vi "_FPGA_Driver_DIO_v1_3.vi"(10 "DO":u8) -> (2 "DI":u8)   [LabVIEW 2018]
uses:
  <vilib>/rvi/eio/common/nirviEmuTemplateMethod_errors.vi
  <vilib>/eio/EIONode/EIONode.xnode
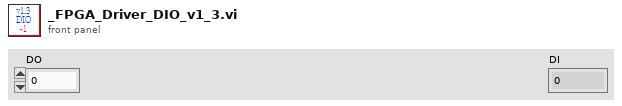
[diagram p1: front panel]
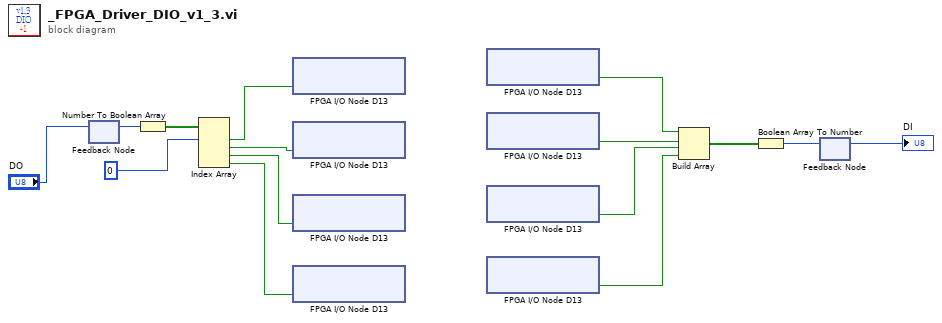
[diagram p0: block diagram]
diagram:
  n1 = feedback-in #1("DO") -> ()
  n2 = feedback #1() -> (w10:u8)  [unwired: 1 in]
  n3 = Number To Boolean Array(number=w10) -> (Boolean array=w14:bool[])
  n4 = Index Array(array=w14, index #1=0 ("index")) -> (element #1=w8:bool, element #2=w7:bool, element #3=w6:bool, element #4=w5:bool)  [unwired: 3 in]
  n5 = xnode "FPGA I/O Node D13"("RMC/DIO20"=w8) -> ()  [unwired: 1 in, 1 out]
  n6 = xnode "FPGA I/O Node D13"("RMC/DIO51"=w7) -> ()  [unwired: 1 in, 1 out]
  n7 = xnode "FPGA I/O Node D13"("RMC/DIO83"=w6) -> ()  [unwired: 1 in, 1 out]
  n8 = xnode "FPGA I/O Node D13"("RMC/DIO18"=w5) -> ()  [unwired: 1 in, 1 out]
  n9 = xnode "FPGA I/O Node D13"() -> ("RMC/DIO24"=w4:bool)  [unwired: 1 in, 1 out]
  n10 = xnode "FPGA I/O Node D13"() -> ("RMC/DIO22"=w3:bool)  [unwired: 1 in, 1 out]
  n11 = xnode "FPGA I/O Node D13"() -> ("RMC/DIO53"=w2:bool)  [unwired: 1 in, 1 out]
  n12 = xnode "FPGA I/O Node D13"() -> ("RMC/DIO85"=w1:bool)  [unwired: 1 in, 1 out]
  n13 = Build Array(w4, w3, w2, w1) -> (w12:bool[])
  n14 = Boolean Array To Number(Boolean array=w12) -> (number=w11:u8)
  n15 = feedback-in #2(w11) -> ()
  n16 = feedback #2() -> (→"DI":u8)  [unwired: 1 in]
